vi "VNAviewer.vi"() -> ()   [LabVIEW 2013]
panel:
  in  "stop":bool
  out "XY Graph":cluster{dbl[], dbl[]}(graph)
  in  "Start Freq":dbl=1700.0
  in  "Stop Freq":dbl=2600.0
  in  "# of points":i32=401
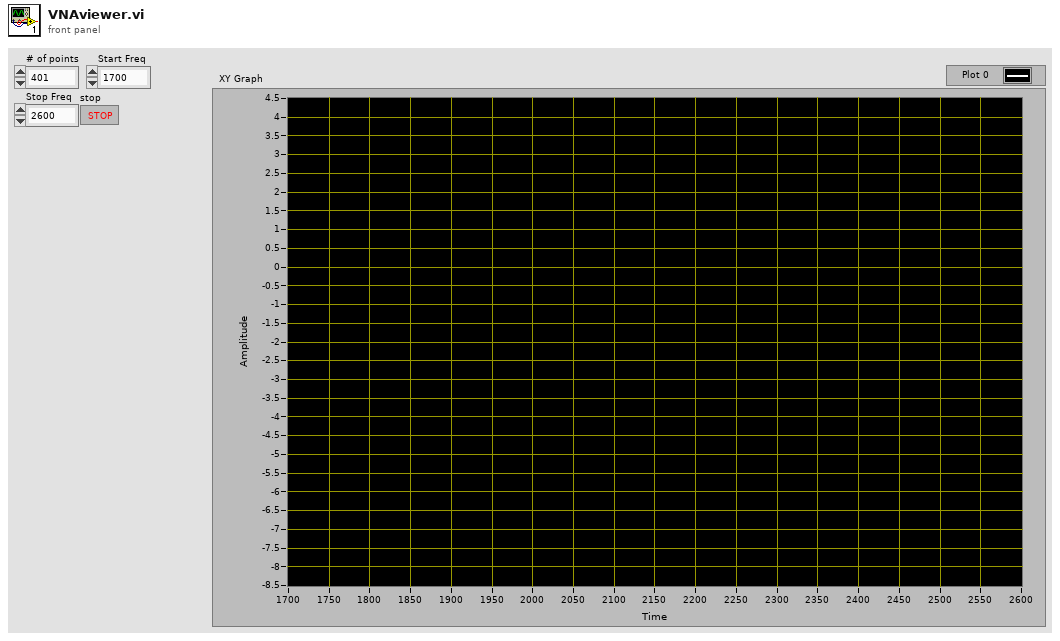
[diagram p1: front panel]
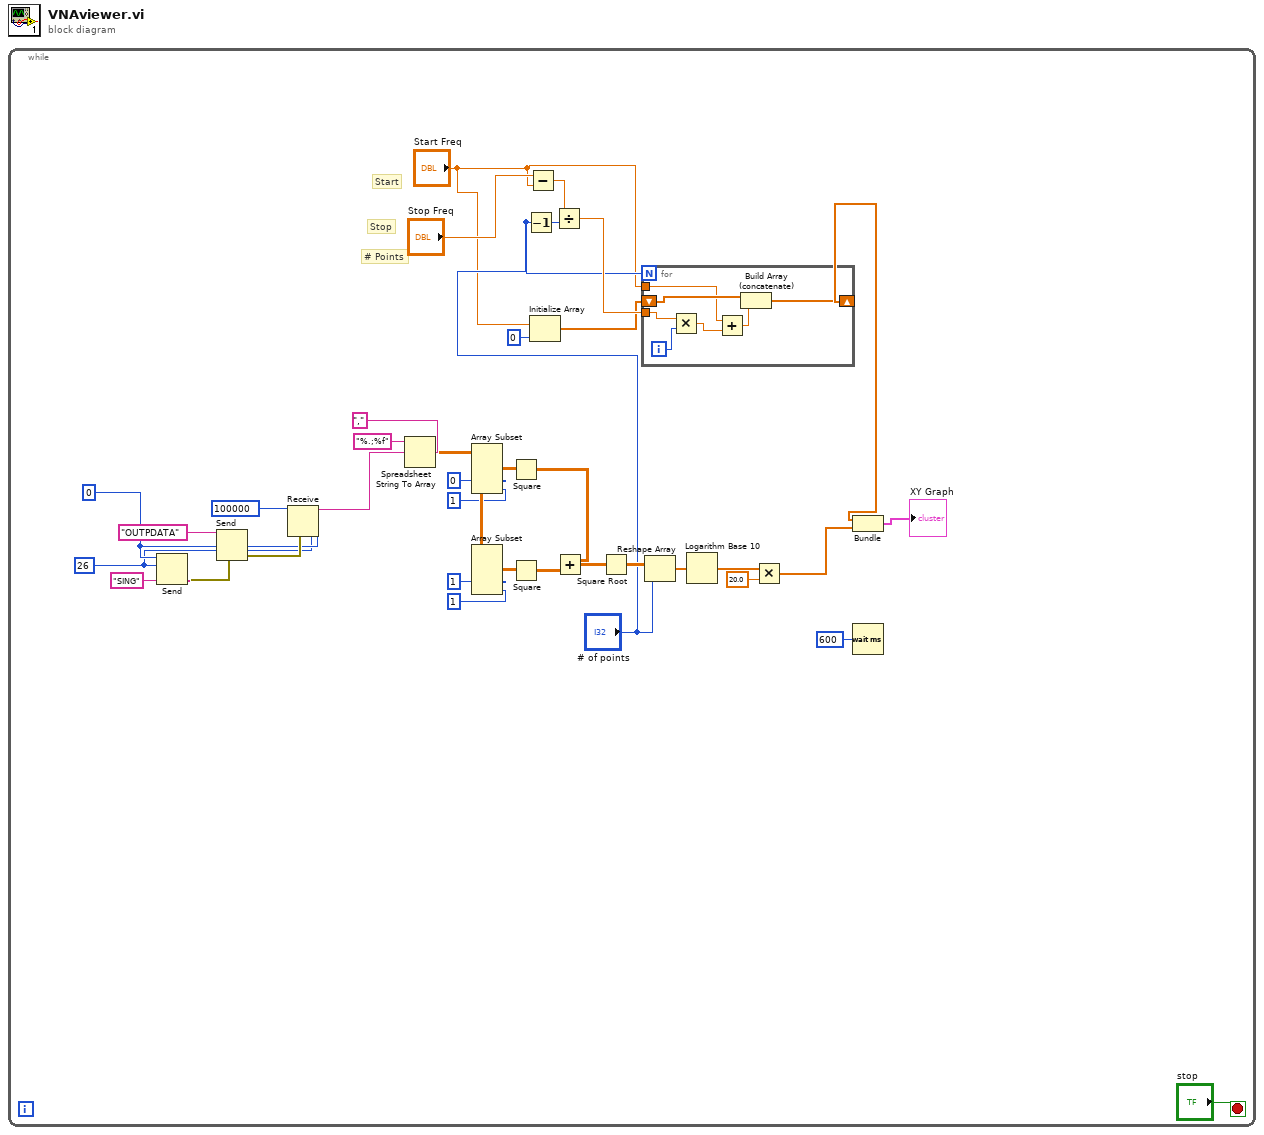
[diagram p0: block diagram]
diagram:
  n1 = while {
    stop <- "stop" stop-if-true
    w14 = i16 26 ("address")
    w15 = 0 ("bus")
    # "# Points"
    # "Stop"
    # "Start"
    n2 = Send(0:w15, 2:w14, 5:"SING" ("data string")) -> (8:w35:errorcluster)  [unwired: 2 in, 2 out]
    n3 = Send(0:w15, 2:w14, 4:w35, 5:"OUTPDATA" ("data string")) -> (8:w34:errorcluster)  [unwired: 1 in, 2 out]
    n4 = Receive(4:w34, 6:100000 ("byte count"), 8:w14, 9:w15) -> (3:w32:string)  [unwired: 1 in, 3 out]
    n5 = Spreadsheet String To Array(delimiter (Tab)=",", format string="%.;%f", spreadsheet string=w32) -> (array=w29:dbl[][])  [unwired: 1 in]
    n6 = Array Subset(array=w29, index (col)=0 ("index"), length (col)=1 ("length")) -> (w24:dbl[][])  [unwired: 2 in]
    n7 = Array Subset(array=w29, index (col)=1 ("index"), length (col)=1 ("length")) -> (w23:dbl[][])  [unwired: 2 in]
    n8 = Square(x=w24) -> (x^2=w21:dbl[][])
    n9 = Square(x=w23) -> (x^2=w22:dbl[][])
    n10 = Decrement(x="# of points") -> (x-1=w13:i32)
    n11 = Subtract(x="Stop Freq", y="Start Freq") -> (x-y=w6:dbl)
    n12 = Initialize Array("Start Freq", 0 ("dimension size")) -> (w10:dbl[])
    n13 = Divide(x=w6, y=w13) -> (x/y=w12:dbl)
    n14 = Add(x=w21, y=w22) -> (x+y=w20:dbl[][])
    n15 = Square Root(x=w20) -> (sqrt(x)=w19:dbl[][])
    n16 = for {
      N: "# of points" -> [_]
      shift-right: [w43] -> w8
      shift-left: w10 -> [w44]
      tunnel: w12 -> [w40]
      tunnel: "Start Freq" -> [w41]
      i -> [w39]
      n17 = Multiply(x=w40, y=w39) -> (x*y=w38:dbl)
      n18 = Add(x=w41, y=w38) -> (x+y=w42:dbl)
      n19 = Build Array (concatenate)(w44, w42) -> (w43:dbl[])
    }
    n20 = Reshape Array(w19, "# of points") -> (w18:dbl[])
    n21 = Logarithm Base 10(1:w18) -> (0:w16:dbl[])
    n22 = Multiply(x=w16, y=20.0) -> (x*y=w17:dbl[])
    n23 = Bundle(w8, w17) -> (→"XY Graph":cluster{dbl[], dbl[]})  [unwired: 1 in]
    n24 = Wait (ms)(milliseconds to wait=u32 600) -> ()  [unwired: 1 out]
  }
